vi "AWS-S3-SendProgressUpdate.vi"(4 "TotalBytes":i64, 5 "Initial Timestamp":u32, 6 "TransferredBytes":i64, 7 "Time Stamp":u32, 8 "Local Filepath":path, 9 "Key":string, 10 "BucketName":string, 11 "User Event in":refnum<user-event>) -> ()   [LabVIEW 2012, in "AWS-S3-API.lvclass"]
uses:
  AWS-S3-API.lvclass
  AWS-S3-Transfer-Progress.ctl
  AWS-S3-Transfer-Header.ctl
panel:
  # "Inputs"
  # "Outputs"
  # "No Outputs - this VI\nis fire and forget"
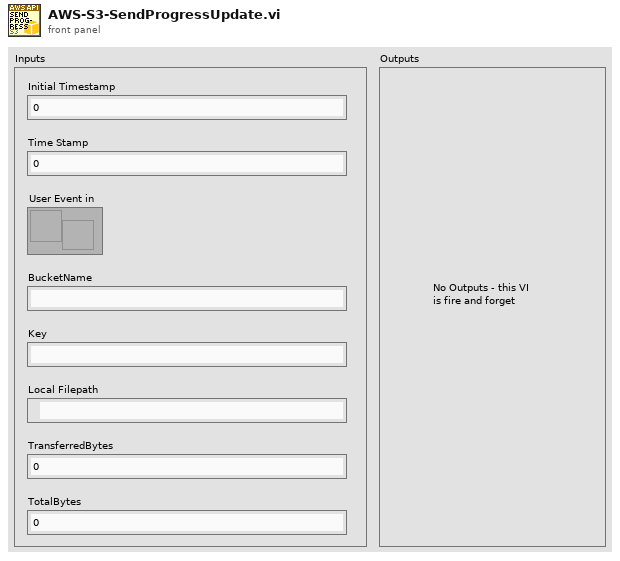
[diagram p1: front panel]
types:
  T1 = typedef "AWS-S3-API.lvclass/AWS-S3-Transfer-Progress.ctl" = cluster{"Transfer Header":T2, "Total Bytes":i64, "Transferred Bytes":i64, "Total MB":dbl, "Transferred MB":dbl, "Percent Done (0.0-100.0%)":dbl, "Current Rate (kB/sec)":dbl, "Time Elapsed (sec)":i32, "Est. Time Remaining (sec)":i32}
  T2 = typedef "AWS-S3-API.lvclass/AWS-S3-Transfer-Header.ctl" = cluster{"Bucket Name":string, "Object Name":string, "Local Filepath":path}
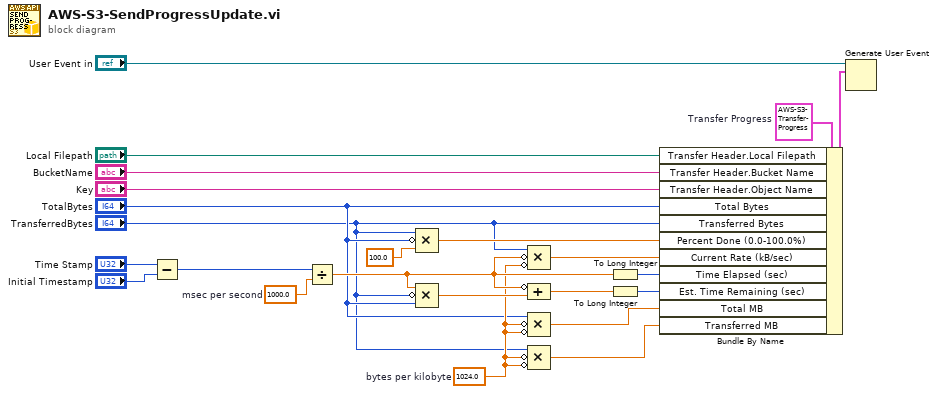
[diagram p0: block diagram]
diagram:
  w19 = 1000.0  # msec per second
  w3 = 1024.0  # bytes per kilobyte
  w12 = T1 {"Transfer Header"={"Bucket Name"="", "Object Name"="", "Local Filepath"=path ""}, "Total Bytes"=0, "Transferred Bytes"=0, "Total MB"=0.0, "Transferred MB"=0.0, "Percent Done (0.0-100.0%)"=0.0, "Current Rate (kB/sec)"=0.0, "Time Elapsed (sec)"=0, "Est. Time Remaining (sec)"=0}  # Transfer Progress
  n1 = Subtract(x="Time Stamp", y="Initial Timestamp") -> (x-y=w18:u32)
  n2 = Divide(x=w18, y=w19) -> (x/y=w20:dbl)
  n3 = Compound Arithmetic op=MULTIPLY("TransferredBytes", invert "TotalBytes", 100.0 ("value")) -> (w13:dbl)
  n4 = Compound Arithmetic op=MULTIPLY(w20, invert "TransferredBytes", "TotalBytes") -> (w16:dbl)
  n5 = Compound Arithmetic op=MULTIPLY("TransferredBytes", invert w20, invert w3) -> (w15:dbl)
  n6 = Compound Arithmetic op=ADD(invert w20, w16) -> (w17:dbl)
  n7 = Compound Arithmetic op=MULTIPLY("TotalBytes", invert w3, invert w3) -> (w5:dbl)
  n8 = Compound Arithmetic op=MULTIPLY("TransferredBytes", invert w3, invert w3) -> (w4:dbl)
  n9 = To Long Integer(number=w20) -> (32bit integer=w21:i32)
  n10 = To Long Integer(number=w17) -> (32bit integer=w22:i32)
  n11 = Bundle By Name(cluster=w12, "Transfer Header.Local Filepath"="Local Filepath", "Transfer Header.Bucket Name"="BucketName", "Transfer Header.Object Name"="Key", "Total Bytes"="TotalBytes", "Transferred Bytes"="TransferredBytes", "Percent Done (0.0-100.0%)"=w13, "Current Rate (kB/sec)"=w15, "Time Elapsed (sec)"=w21, "Est. Time Remaining (sec)"=w22, "Total MB"=w5, "Transferred MB"=w4) -> (w11:T1)
  n12 = Generate User Event(user event="User Event in", event data cluster=w11) -> ()  [unwired: 1 in, 2 out]
